vi "Convert Message.vi"(8 "error in (no error)":errorcluster, 11 "Engine RPM in":refnum<class "VIN.lvclass">) -> (0 "error out":errorcluster, 1 "variant":variant, 2 "Result":dbl, 3 "Engine RPM out":refnum<class "VIN.lvclass">)   [LabVIEW 2011, in "VIN.lvclass"]
uses:
  VIN.lvclass
  PID.lvclass
panel:
  out "VIN":string
  out "concatenated string":string
  out "Line 2":string
  out "Line 1":string
  out "Line 0":string
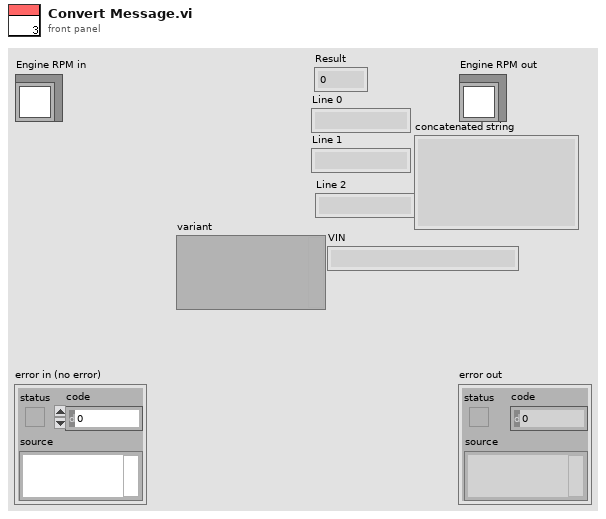
[diagram p1: front panel]
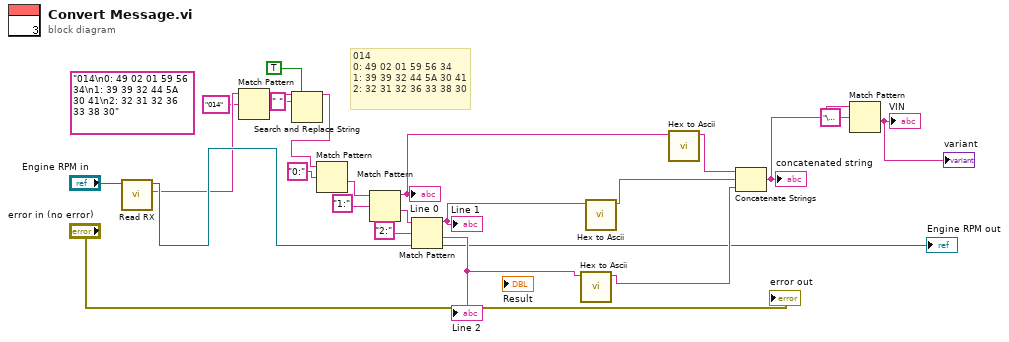
[diagram p0: block diagram]
diagram:
  (unwired) "014\n0: 49 02 01 59 56 34\n1: 39 39 32 44 5A 30 41\n2: 32 31 32 36 33 38 30" ("Response In")
  # "014\n0: 49 02 01 59 56 34\n1: 39 39 32 44 5A 30 41\n2: 32 31 32 36 33 38 30"
  n1 = call "Read RX.vi"("PID in"="Engine RPM in") -> ("RX"=w6:string, "PID out"=→"Engine RPM out":refnum<class "VIN.lvclass">)  [unwired: 8 in, 1 out]
  n2 = Match Pattern(string=w6, regular expression="014") -> (after substring=w4:string)  [unwired: 1 in, 3 out]
  n3 = Search and Replace String(replace all?=TRUE ("replace all? (F)"), input string=w4, search string=" ") -> (result string=w2:string)  [unwired: 5 in, 3 out]
  n4 = Match Pattern(string=w2, regular expression="0:" ("search string")) -> (after substring=w20:string)  [unwired: 1 in, 3 out]
  n5 = Match Pattern(string=w20, regular expression="1:" ("search string")) -> (before substring=w16:string, after substring=w17:string)  [unwired: 1 in, 2 out]
  "Line 0" <- w16
  n6 = Match Pattern(string=w17, regular expression="2:" ("search string")) -> (before substring=w15:string, after substring=w14:string)  [unwired: 1 in, 2 out]
  "Line 1" <- w15
  "Line 2" <- w14
  n7 = call "Hex to Ascii.vi"("result string"=w14) -> ("String"=w11:string)  [unwired: 9 in, 1 out]
  n8 = call "Hex to Ascii.vi"("result string"=w15) -> ("String"=w12:string)  [unwired: 9 in, 1 out]
  n9 = call "Hex to Ascii.vi"("result string"=w16) -> ("String"=w13:string)  [unwired: 9 in, 1 out]
  n10 = Concatenate Strings(w13, w12, w11) -> (w10:string)
  "concatenated string" <- w10
  n11 = Match Pattern(string=w10, regular expression="\u0001") -> (after substring=→"variant" →"VIN":string)  [unwired: 1 in, 3 out]
  "error out" <- "error in (no error)"
